vi "Assign Value.vi"(8 "error in (no error)":errorcluster, 10 "Assigned Value":refnum<class "Abs_Value.lvclass">, 11 "Abs_Double Float in":refnum<class "Abs_Double Float.lvclass">) -> (0 "error out":errorcluster, 3 "Abs_Double Float out":refnum<class "Abs_Double Float.lvclass">)   [LabVIEW 2021, in "Abs_Double Float.lvclass"]
uses:
  Abs_Double Float.lvclass
  Value/Abs_Value.lvclass
  Numeric/Abs_Numeric.lvclass
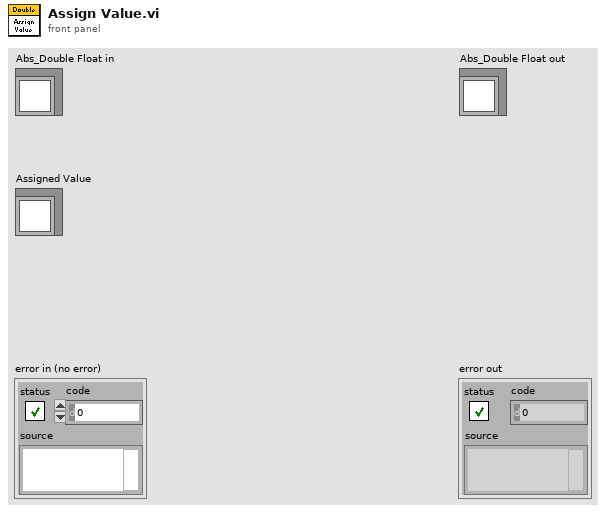
[diagram p1: front panel]
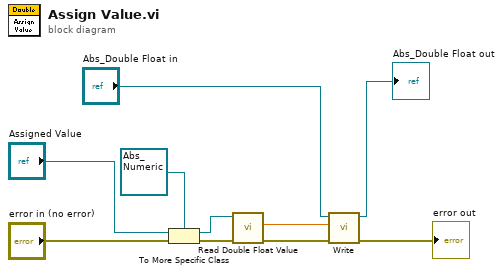
[diagram p0: block diagram]
diagram:
  n1 = To More Specific Class(target class=refnum<class "Abs_Numeric.lvclass"> refnum ("Abs_Numeric.lvclass"), reference="Assigned Value", error in="error in (no error)") -> (specific class reference=w3:refnum<class "Abs_Numeric.lvclass">, error out=w5:errorcluster)
  n2 = call-dynamic "Read Double Float Value.vi"("error in (no error)"=w5, "Numeric in"=w3) -> ("error out"=w2:errorcluster, "Double"=w1:dbl)  [unwired: 7 in, 1 out]
  n3 = call-dynamic "Write.vi"("error in (no error)"=w2, "Value"=w1, "Double Float.lvclass in"="Abs_Double Float in") -> ("error out"=→"error out":errorcluster, "Double Float.lvclass out"=→"Abs_Double Float out":refnum<class "Abs_Double Float.lvclass">)  [unwired: 7 in]
